vi "CommandFIFOMultiplexer.vi"   [LabVIEW 2016]
uses:
  <vilib>/rvi/Emulation/niFpgaGetClockAttributes.vi
  <vilib>/rvi/Emulation/niFpgaSctlEmulationGetInTimedLoop.vi
  <vilib>/rvi/Emulation/niFpgaEmulationReportErrorSimple.vi
  <vilib>/rvi/interface/RandomDataEmulation/niFpgaRandomDataHandleErrors.vi
  <vilib>/rvi/Emulation/niFpgaEmulationIsFPGAContextNoSignature.vi
  <vilib>/rvi/errors/niFpgaSetErrorForExecOnDevCompSimple.vi
  <vilib>/rvi/eio/common/nirviEmuReportErrorAndStop.vi
  <vilib>/rvi/DataTransferAndStorage/Container/Common/niFpgaContainerGetUniqueNameForEmu.vi
  <vilib>/rvi/FIFO/Fifo_Resource/nirvififoEmulationSetSize.vi
  <vilib>/rvi/FIFO/Fifo_Resource/nirviFifoEmulationQueueMgr.vi
  <instcachedir>/0/nirviFifoEmulationQueueMgr_E5CAEC123FF24DC58D834DCA3CDAA9B5.lvgen/nirviFifoEmulationQueueMgr_E5CAEC123FF24DC58D834DCA3CDAA9B5_007.vi
  <vilib>/rvi/FIFO/Fifo_Resource/nirvififoEmulationDetermineInputValidOut.vi
  <vilib>/rvi/FIFO/Fifo_Resource/nirvififoEmulationCreateLock.vi
  <vilib>/rvi/Emulation/niFpgaProcessEmulError.vi
  <vilib>/rvi/FIFO/Fifo_Resource/nirvififoEmulationObtainLock.vi
  <vilib>/rvi/FIFO/Fifo_Resource/nirvififoEmulationReleaseLock.vi
  <vilib>/rvi/occurrence/nirviWaitOnOccurrenceBase.vi
  <vilib>/rvi/errors/nirviReportUnexpectedCaseInternalError.vi
  <vilib>/rvi/errors/nirviReportUnexpectedCaseInternalError (U32).vi
  <vilib>/rvi/Memory/Memory_Emulation/niFpgaMemoryEmulationCacheClearOnFirstRun.vi
  <vilib>/rvi/Memory/Memory_Emulation/nirvimemoryEmulationManagerCache_MakeExclusive.vi
  <vilib>/rvi/Memory/Memory_Emulation/niFpgaMemoryEmulationValidateCache.vi
  <vilib>/rvi/Memory/Memory_Emulation/nirvimemoryEmulationManagerCache_InsertValue.vi
  <vilib>/Utility/error.llb/Clear Errors.vi
  <vilib>/rvi/Memory/Memory_Emulation/nirvimemoryEmulationManagerCache_ReleaseExclusive.vi
  <vilib>/rvi/Memory/Memory_Emulation/nirvimemoryEmulationManagerCache_GetValue.vi
  <vilib>/rvi/Memory/Memory_Emulation/nirvimemoryEmulationManagerCache_SetValue.vi
  <vilib>/rvi/Emulation/niFpgaCriticalErrorInLSC.vi
  <vilib>/rvi/DataTransferAndStorage/Container/XNode/niFpgaContainer.xnode
  <vilib>/rvi/interface/RandomDataEmulation/nirviRandomDataFpgaReadWriteTemplate.vi
  <vilib>/rvi/FIFO/Fifo_Resource/nirvififoEmulationWrite.vi
  <vilib>/rvi/DataTransferAndStorage/Register/Emulation/niFpgaRegisterEmulation.vi
types:
  T1 = typedef "Addresses.ctl" = enum8{"NA", "Slot1/AI0-AccelerometerAx", "Slot1/AI1-AccelerometerAz", "Slot1/AI2-AccelerometerBy", "Slot1/AI3-AccelerometerBz", "Slot2/AI0-AccelerometerCx", "Slot2/AI1-AccelerometerCz", "Slot2/AI2-AccelerometerDy", "Slot2/AI3-AccelerometerDz", "Slot3/DIO0-ModbusSubnetATx", "Slot3/DIO1-ModbusSubnetBTx", "Slot3/DIO2-ModbusSubnetCTx", "Slot3/DIO3-ModbusSubnetDTx", "Slot3/DIO4-ModbusSubnetARx", "Slot3/DIO5-ModbusSubnetBRx", "Slot3/DIO6-ModbusSubnetCRx", "Slot3/DIO7-ModbusSubnetDRx", "Slot4/DIO0-ModbusSubnetETx", "Slot4/DIO1-GyroTx", "Slot4/DIO2", "Slot4/DIO3", "Slot4/DIO4-ModbusSubnetERx", "Slot4/DIO5-GyroRx", "Slot4/DIO6", "Slot4/DIO7", "Slot5/DI0-ILCPowerInterlockStatus", "Slot5/DI1-FanCoilHeaterInterlockStatus", "Slot5/DI2-LaserTrackerInterlockStatus", "Slot5/DI3-AirSupplyInterlockStatus", "Slot5/DI4-GISEarthquakeInterlockStatus", "Slot5/DI5-GISEStopInterlockStatus", "Slot5/DI6-TMAMotionStopInterlockStatus", "Slot5/DI7-GISHeartbeatInterlockStatus", "Slot5/DI8-AirSupplyValveOpen", "Slot5/DI9-AirSupplyValveClosed", "Slot5/DI10-MirrorCellLightsOn", "Slot5/DI11", "Slot5/DI12", "Slot5/DI13", "Slot5/DI14", "Slot5/DI15", "Slot5/DO0", "Slot5/DO1", "Slot5/DO2", "Slot5/DO3", "Slot5/DO4", "Slot5/DO5", "Slot5/DO6", "Slot5/DO7", "Slot5/DO8", "Slot5/DO9", "Slot5/DO10", "Slot5/DO11", "Slot5/DO12", "Slot5/DO13", "Slot5/DO14", "Slot5/DO15", "Slot6/CH0-HeartbeatToSafetyController", "Slot6/CH1-CriticalFaultToSafetyController", "Slot6/CH2-MirrorLoweringRaisingToSafetyController", "Slot6/CH3-MirrorParkedToSafetyController", "Slot6/CH4-AirSupplyValveControl", "Slot6/CH5-MirrorCellLightControl", "Slot6/CH6", "Slot6/CH7", "Slot7/CH0-AuxPowerNetworkAOn", "Slot7/CH1-AuxPowerNetworkBOn", "Slot7/CH2-AuxPowerNetworkCOn", "Slot7/CH3-AuxPowerNetworkDOn", "Slot7/CH4-PowerNetworkAOn", "Slot7/CH5-PowerNetworkBOn", "Slot7/CH6-PowerNetworkCOn", "Slot7/CH7-PowerNetworkDOn", "Slot8/Port1-Displacement", "Slot8/Port2-Inclinometer", "Slot8/Port3", "Slot8/Port4", "Undefined1", "Undefined2", "Undefined3", "Undefined4", "Undefined5", "Undefined6", "Undefined7", "Undefined8", "Undefined9", "Undefined10", "Undefined11", "Undefined12", "Undefined13", "Undefined14", "Undefined15", "Undefined16", "Undefined17", "Undefined18", "Undefined19", "Undefined20", "Undefined21", "Undefined22", "Undefined23", "Undefined24", "Undefined25", "Undefined26", "Undefined27", "Undefined28", "Undefined29", "Undefined30", "Undefined31", "Undefined32", "Undefined33", "Undefined34", "Undefined35", "Undefined36", "Undefined37", "Undefined38", "Undefined39", "Undefined40", "Undefined41", "Undefined42", "Undefined43", "Undefined44", "Undefined45", "Undefined46", "Undefined47", "Undefined48", "Undefined49", "Undefined50", "Undefined51", "Undefined52", "Undefined53", "Undefined54", "Undefined55", "Undefined56", "Undefined57", "Undefined58", "Undefined59", "Undefined60", "Undefined61", "Undefined62", "Undefined63", "Undefined64", "Undefined65", "Undefined66", "Undefined67", "Undefined68", "Undefined69", "Undefined70", "Undefined71", "Undefined72", "Undefined73", "Undefined74", "Undefined75", "Undefined76", "Undefined77", "Undefined78", "Undefined79", "Undefined80", "Undefined81", "Undefined82", "Undefined83", "Undefined84", "Undefined85", "Undefined86", "Undefined87", "Undefined88", "Undefined89", "Undefined90", "Undefined91", "Undefined92", "Undefined93", "Undefined94", "Undefined95", "Undefined96", "Undefined97", "Undefined98", "Undefined99", "Undefined100", "Undefined101", "Undefined102", "Undefined103", "Undefined104", "Undefined105", "Undefined106", "Undefined107", "Undefined108", "Undefined109", "Undefined110", "Undefined111", "Undefined112", "Undefined113", "Undefined114", "Undefined115", "Undefined116", "Undefined117", "Undefined118", "Undefined119", "Undefined120", "Undefined121", "Undefined122", "Undefined123", "Undefined124", "Undefined125", "Undefined126", "Undefined127", "Undefined128", "Undefined129", "Undefined130", "Undefined131", "Undefined132", "Undefined133", "Undefined134", "Undefined135", "Undefined136", "Undefined137", "Undefined138", "Undefined139", "Undefined140", "Undefined141", "Undefined142", "Undefined143", "Undefined144", "Undefined145", "Undefined146", "Undefined147", "Undefined148", "Undefined149", "Undefined150", "Undefined151", "Undefined152", "Undefined153", "Undefined154", "Undefined155", "Undefined156", "Undefined157", "Undefined158", "Undefined159", "Undefined160", "Undefined161", "Undefined162", "Undefined163", "Undefined164", "Undefined165", "Undefined166", "Undefined167", "Undefined168", "Undefined169", "Undefined170", "Undefined171", "Undefined172", "Undefined173", "Undefined174", "GyroRxIgnore", "ModbusSoftwareTrigger", "Accelerometers", "HealthAndStatus", "Timestamp"}
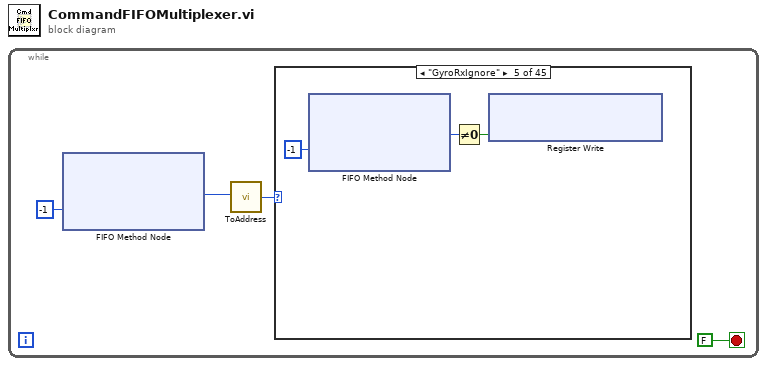
[diagram p0: block diagram]
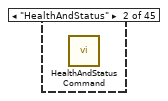
[diagram p3: hidden frame]
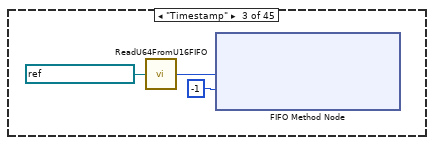
[diagram p4: hidden frame]
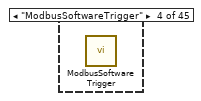
[diagram p5: hidden frame]
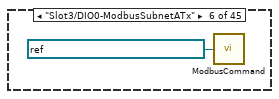
[diagram p6: hidden frame]
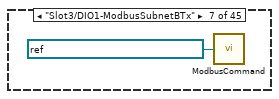
[diagram p7: hidden frame]
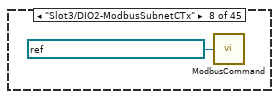
[diagram p8: hidden frame]
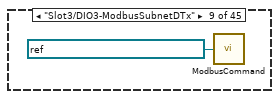
[diagram p9: hidden frame]
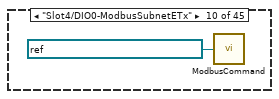
[diagram p10: hidden frame]
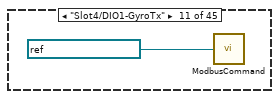
[diagram p11: hidden frame]
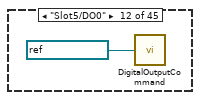
[diagram p12: hidden frame]
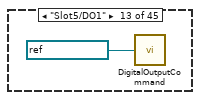
[diagram p13: hidden frame]
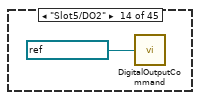
[diagram p14: hidden frame]
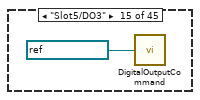
[diagram p15: hidden frame]
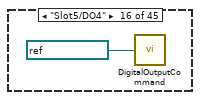
[diagram p16: hidden frame]
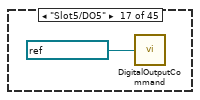
[diagram p17: hidden frame]
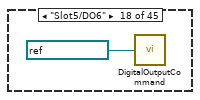
[diagram p18: hidden frame]
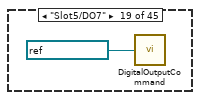
[diagram p19: hidden frame]
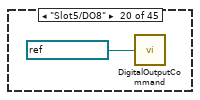
[diagram p20: hidden frame]
diagram:
  n1 = while {
    stop <- FALSE stop-if-true
    n2 = xnode ("FIFO Method Node")("Timeout"=-1) -> ("Element"=w3:u16)  [unwired: 1 in, 2 out]
    n3 = call "ToAddress.vi"("Input"=w3) -> ("Address"=w2:T1)
    n4 = case shown="\"GyroRxIgnore\"" w2 {
      frame "NA", Default {
      }
      frame "HealthAndStatus" {
        n5 = call "HealthAndStatusCommand.vi"() -> ()  [unwired: 12 in]
      }
      frame "Timestamp" {
        n6 = call "ReadU64FromU16FIFO.vi"("FIFO In"=refnum<k21> "CommandFIFO") -> ("U64"=w6:u64)
        n7 = xnode ("FIFO Method Node")("Element"=w6, "Timeout"=-1) -> ()  [unwired: 1 in, 2 out]
      }
      frame "ModbusSoftwareTrigger" {
        n8 = call "ModbusSoftwareTrigger.vi"() -> ()  [unwired: 12 in]
      }
      frame "GyroRxIgnore" {
        n9 = xnode ("FIFO Method Node")("Timeout"=-1) -> ("Element"=w8:u16)  [unwired: 1 in, 2 out]
        n10 = Not Equal To 0?(x=w8) -> (x != 0?=w10:bool)
        n11 = xnode "Register Write"("Data"=w10) -> ()  [unwired: 1 in, 1 out]
      }
      frame "Slot3/DIO0-ModbusSubnetATx" {
        n12 = call "ModbusCommand.vi"("SubnetTxFIFO"=refnum<k21> "ModbusSubnetATxDataFIFO") -> ()  [unwired: 1 in]
      }
      frame "Slot3/DIO1-ModbusSubnetBTx" {
        n13 = call "ModbusCommand.vi"("SubnetTxFIFO"=refnum<k21> "ModbusSubnetBTxDataFIFO") -> ()  [unwired: 1 in]
      }
      frame "Slot3/DIO2-ModbusSubnetCTx" {
        n14 = call "ModbusCommand.vi"("SubnetTxFIFO"=refnum<k21> "ModbusSubnetCTxDataFIFO") -> ()  [unwired: 1 in]
      }
      frame "Slot3/DIO3-ModbusSubnetDTx" {
        n15 = call "ModbusCommand.vi"("SubnetTxFIFO"=refnum<k21> "ModbusSubnetDTxDataFIFO") -> ()  [unwired: 1 in]
      }
      frame "Slot4/DIO0-ModbusSubnetETx" {
        n16 = call "ModbusCommand.vi"("SubnetTxFIFO"=refnum<k21> "ModbusSubnetETxDataFIFO") -> ()  [unwired: 1 in]
      }
      frame "Slot4/DIO1-GyroTx" {
        n17 = call "ModbusCommand.vi"("SubnetTxFIFO"=refnum<k21> "GyroTxDataFIFO") -> ()  [unwired: 1 in]
      }
      frame "Slot5/DO0" {
        n18 = call "DigitalOutputCommand.vi"("FPGA I/O In"=refnum<k21> "Slot5/DO0") -> ()  [unwired: 1 in]
      }
      frame "Slot5/DO1" {
        n19 = call "DigitalOutputCommand.vi"("FPGA I/O In"=refnum<k21> "Slot5/DO1") -> ()  [unwired: 1 in]
      }
      frame "Slot5/DO2" {
        n20 = call "DigitalOutputCommand.vi"("FPGA I/O In"=refnum<k21> "Slot5/DO2") -> ()  [unwired: 1 in]
      }
      frame "Slot5/DO3" {
        n21 = call "DigitalOutputCommand.vi"("FPGA I/O In"=refnum<k21> "Slot5/DO3") -> ()  [unwired: 1 in]
      }
      frame "Slot5/DO4" {
        n22 = call "DigitalOutputCommand.vi"("FPGA I/O In"=refnum<k21> "Slot5/DO4") -> ()  [unwired: 1 in]
      }
      frame "Slot5/DO5" {
        n23 = call "DigitalOutputCommand.vi"("FPGA I/O In"=refnum<k21> "Slot5/DO5") -> ()  [unwired: 1 in]
      }
      frame "Slot5/DO6" {
        n24 = call "DigitalOutputCommand.vi"("FPGA I/O In"=refnum<k21> "Slot5/DO6") -> ()  [unwired: 1 in]
      }
      frame "Slot5/DO7" {
        n25 = call "DigitalOutputCommand.vi"("FPGA I/O In"=refnum<k21> "Slot5/DO7") -> ()  [unwired: 1 in]
      }
      frame "Slot5/DO8" {
        n26 = call "DigitalOutputCommand.vi"("FPGA I/O In"=refnum<k21> "Slot5/DO8") -> ()  [unwired: 1 in]
      }
      frame "Slot5/DO9" {
        n27 = call "DigitalOutputCommand.vi"("FPGA I/O In"=refnum<k21> "Slot5/DO9") -> ()  [unwired: 1 in]
      }
      frame "Slot5/DO10" {
        n28 = call "DigitalOutputCommand.vi"("FPGA I/O In"=refnum<k21> "Slot5/DO10") -> ()  [unwired: 1 in]
      }
      frame "Slot5/DO11" {
        n29 = call "DigitalOutputCommand.vi"("FPGA I/O In"=refnum<k21> "Slot5/DO11") -> ()  [unwired: 1 in]
      }
      frame "Slot5/DO12" {
        n30 = call "DigitalOutputCommand.vi"("FPGA I/O In"=refnum<k21> "Slot5/DO12") -> ()  [unwired: 1 in]
      }
      frame "Slot5/DO13" {
        n31 = call "DigitalOutputCommand.vi"("FPGA I/O In"=refnum<k21> "Slot5/DO13") -> ()  [unwired: 1 in]
      }
      frame "Slot5/DO14" {
        n32 = call "DigitalOutputCommand.vi"("FPGA I/O In"=refnum<k21> "Slot5/DO14") -> ()  [unwired: 1 in]
      }
      frame "Slot5/DO15" {
        n33 = call "DigitalOutputCommand.vi"("FPGA I/O In"=refnum<k21> "Slot5/DO15") -> ()  [unwired: 1 in]
      }
      frame "Slot6/CH0-HeartbeatToSafetyController" {
        n34 = call "DigitalOutputCommand.vi"("FPGA I/O In"=refnum<k21> "Slot6/CH0") -> ()  [unwired: 1 in]
      }
      frame "Slot6/CH1-CriticalFaultToSafetyController" {
        n35 = call "DigitalOutputCommand.vi"("FPGA I/O In"=refnum<k21> "Slot6/CH1") -> ()  [unwired: 1 in]
      }
      frame "Slot6/CH2-MirrorLoweringRaisingToSafetyController" {
        n36 = call "DigitalOutputCommand.vi"("FPGA I/O In"=refnum<k21> "Slot6/CH2") -> ()  [unwired: 1 in]
      }
      frame "Slot6/CH3-MirrorParkedToSafetyController" {
        n37 = call "DigitalOutputCommand.vi"("FPGA I/O In"=refnum<k21> "Slot6/CH3") -> ()  [unwired: 1 in]
      }
      frame "Slot6/CH4-AirSupplyValveControl" {
        n38 = call "DigitalOutputCommand.vi"("FPGA I/O In"=refnum<k21> "Slot6/CH4") -> ()  [unwired: 1 in]
      }
      frame "Slot6/CH5-MirrorCellLightControl" {
        n39 = call "DigitalOutputCommand.vi"("FPGA I/O In"=refnum<k21> "Slot6/CH5") -> ()  [unwired: 1 in]
      }
      frame "Slot6/CH6" {
        n40 = call "DigitalOutputCommand.vi"("FPGA I/O In"=refnum<k21> "Slot6/CH6") -> ()  [unwired: 1 in]
      }
      frame "Slot6/CH7" {
        n41 = call "DigitalOutputCommand.vi"("FPGA I/O In"=refnum<k21> "Slot6/CH7") -> ()  [unwired: 1 in]
      }
      frame "Slot7/CH0-AuxPowerNetworkAOn" {
        n42 = call "DigitalOutputCommand.vi"("FPGA I/O In"=refnum<k21> "Slot7/CH0") -> ()  [unwired: 1 in]
      }
      frame "Slot7/CH1-AuxPowerNetworkBOn" {
        n43 = call "DigitalOutputCommand.vi"("FPGA I/O In"=refnum<k21> "Slot7/CH1") -> ()  [unwired: 1 in]
      }
      frame "Slot7/CH2-AuxPowerNetworkCOn" {
        n44 = call "DigitalOutputCommand.vi"("FPGA I/O In"=refnum<k21> "Slot7/CH2") -> ()  [unwired: 1 in]
      }
      frame "Slot7/CH3-AuxPowerNetworkDOn" {
        n45 = call "DigitalOutputCommand.vi"("FPGA I/O In"=refnum<k21> "Slot7/CH3") -> ()  [unwired: 1 in]
      }
      frame "Slot7/CH4-PowerNetworkAOn" {
        n46 = call "DigitalOutputCommand.vi"("FPGA I/O In"=refnum<k21> "Slot7/CH4") -> ()  [unwired: 1 in]
      }
      frame "Slot7/CH5-PowerNetworkBOn" {
        n47 = call "DigitalOutputCommand.vi"("FPGA I/O In"=refnum<k21> "Slot7/CH5") -> ()  [unwired: 1 in]
      }
      frame "Slot7/CH6-PowerNetworkCOn" {
        n48 = call "DigitalOutputCommand.vi"("FPGA I/O In"=refnum<k21> "Slot7/CH6") -> ()  [unwired: 1 in]
      }
      frame "Slot7/CH7-PowerNetworkDOn" {
        n49 = call "DigitalOutputCommand.vi"("FPGA I/O In"=refnum<k21> "Slot7/CH7") -> ()  [unwired: 1 in]
      }
      frame "Slot8/Port1-Displacement" {
        n50 = call "RS232Command.vi"("OutputFIFO"=refnum<k21> "DisplacementTxFIFO") -> ()  [unwired: 1 in]
      }
      frame "Slot8/Port2-Inclinometer" {
        n51 = call "RS232Command.vi"("OutputFIFO"=refnum<k21> "InclinometerTxFIFO") -> ()  [unwired: 1 in]
      }
    }
  }
